vi "Lock-PID.vi"() -> ()   [LabVIEW 2019]
panel:
  out "Lock PID?":bool
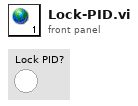
[diagram p1: front panel]
diagram:
